vi "LoadTree2.vi"(8 "error in":errorcluster, 10 "File Path Control":path, 11 "TreeControl reference":refnum<vi>) -> (0 "error out":errorcluster)   [LabVIEW 2014]
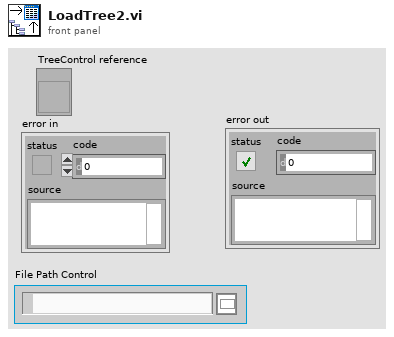
[diagram p1: front panel]
types:
  T1 = cluster{"Left Cell String":string, "Child Text":string[], "Child Tag":string, "Item Indent":i32, "Child Only?":bool, "Glyph Index":i32}[]
  T2 = cluster{"Left Cell String":string, "Child Text":string[], "Child Tag":string, "Item Indent":i32, "Child Only?":bool, "Glyph Index":i32}
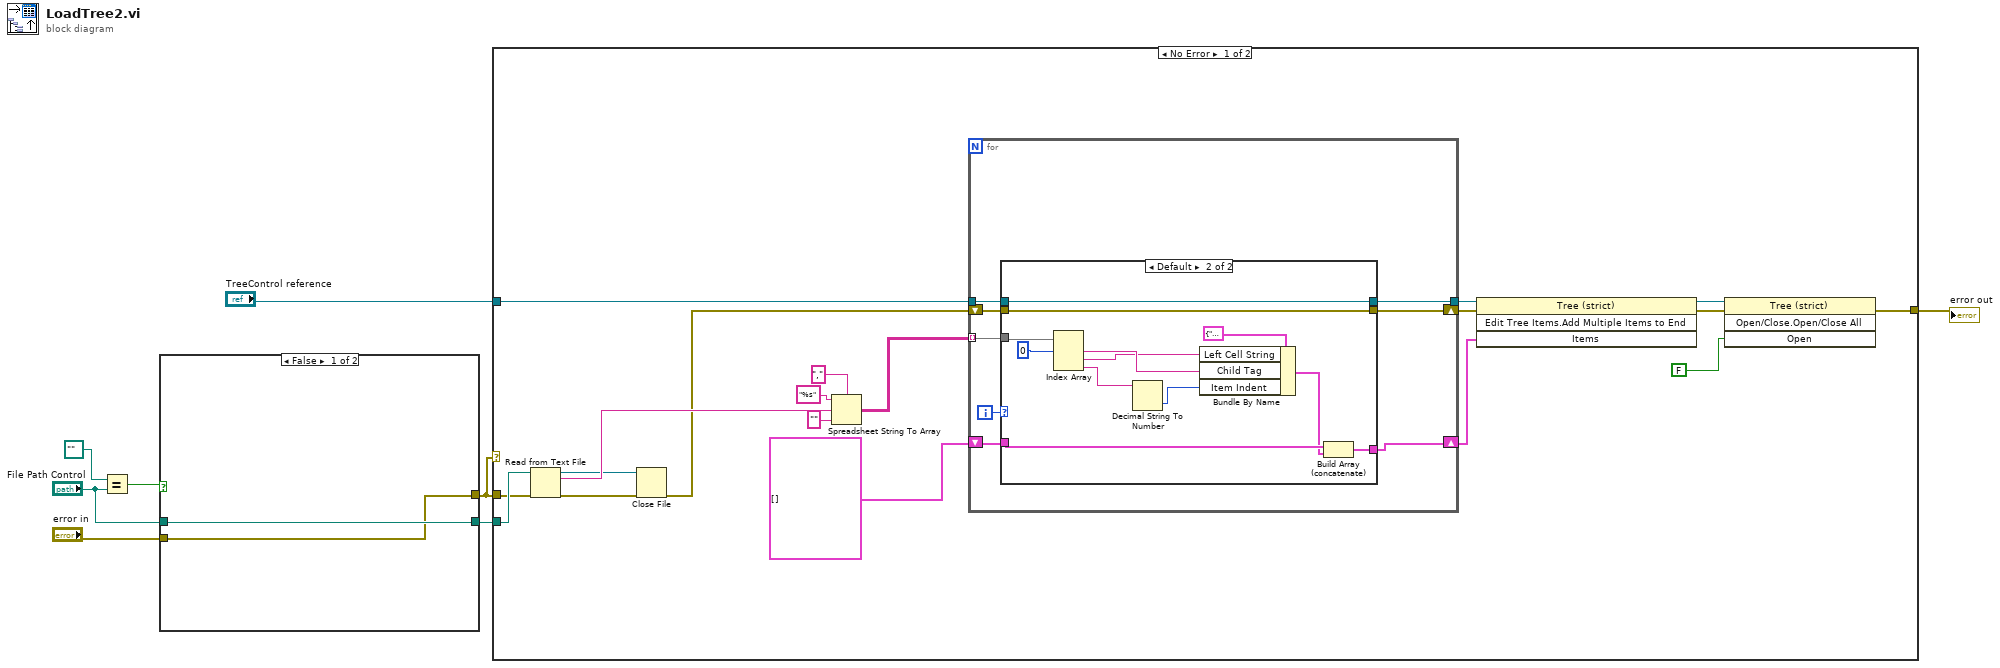
[diagram p0: block diagram]
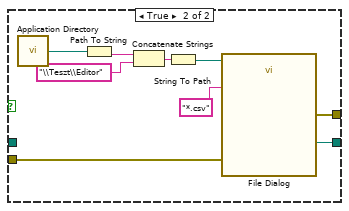
[diagram p2: hidden frame]
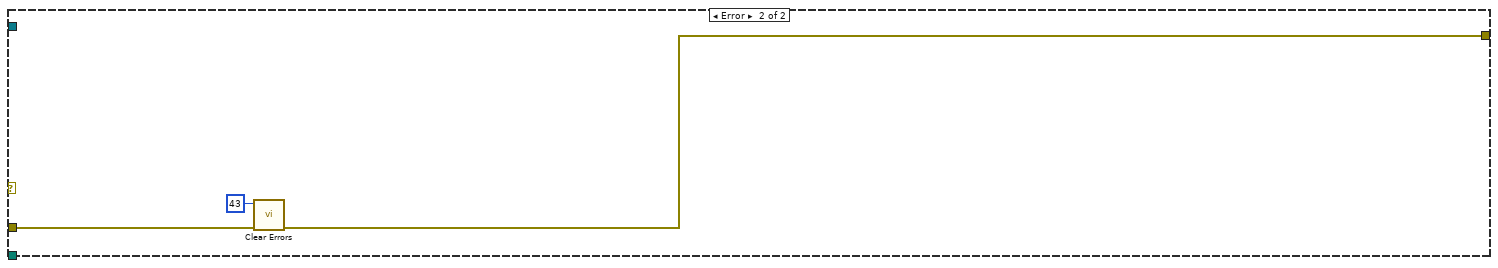
[diagram p4: hidden frame]
diagram:
  n1 = Equal?(x=path "" ("y"), y="File Path Control") -> (x = y?=w3:bool)
  n2 = case shown="False" w3 {
    tunnel: [w10 w13] -> w7
    tunnel: [w9 w12] -> w5
    tunnel: "File Path Control" -> [w10 _]
    tunnel: "error in" -> [w9 w11]
    frame False {
    }
    frame True {
      n3 = call <vilib>:"Application Directory.vi"() -> ("Application Directory"=w14:path)
      n4 = Path To String(path=w14) -> (string=w18:string)
      n5 = Concatenate Strings(w18, "\\Teszt\\Editor" ("prompt (Choose or enter file path)")) -> (w17:string)
      n6 = String To Path(string=w17) -> (path=w15:path)
      n7 = call "File Dialog"("start path"=w15, "error in"=w11, "pattern (all files)"="*.csv") -> ("selected path"=w13:path, "error out"=w12:errorcluster)  [unwired: 9 in, 2 out]
    }
  }
  n8 = case shown="No Error" w5 {
    tunnel: "TreeControl reference" -> [w24 _]
    tunnel: w7 -> [w33 _]
    tunnel: w5 -> [w32 w64]
    tunnel: [w22 w63] -> w6
    frame No Error {
      n9 = Read from Text File(file (use dialog)=w33, error in=w32) -> (refnum out=w36:refnum<file>, text=w37:string, error out=w35:errorcluster)  [unwired: 1 in, 2 out]
      n10 = Close File(refnum=w36, error in=w35) -> (error out=w25:errorcluster)  [unwired: 1 out]
      n11 = Spreadsheet String To Array(delimiter (Tab)=",", format string="%s", spreadsheet string=w37, array type (2D Dbl)="") -> (array=w31:string[][])
      n12 = for {
        tunnel: w24 -> [w46]
        tunnel: w31 -> [w44] mode=indexing
        shift-right: [w45] -> w29
        shift-left: w25 -> [w43]
        tunnel: [w42] -> w30
        shift-right: [w40] -> w27
        shift-left: T1 [] -> [w41]
        i -> [w39]
        n13 = case shown="Default" w39 {
          tunnel: w46 -> [w48 w53]
          tunnel: w43 -> [w49 w54]
          tunnel: [w49 w54] -> w45
          tunnel: w44 -> [_ w59]
          tunnel: [w48 w53] -> w42
          tunnel: w41 -> [w47 w52]
          tunnel: [w47 w50] -> w40
          frame 0 {
            # "fejlécet eldobjuk"
          }
          frame Default {
            n14 = Index Array(array=w59, index #1=0 ("index")) -> (element #1=w56:string, element #2=w55:string, element #3=w60:string)  [unwired: 2 in]
            n15 = Decimal String To Number(string=w60) -> (number=w57:i32)  [unwired: 2 in, 1 out]
            n16 = Bundle By Name(cluster=T2 {"Left Cell String"="Top Level Parent", "Child Text"=[], "Child Tag"="", "Item Indent"=0, "Child Only?"=FALSE, "Glyph Index"=0} ("Item"), "Left Cell String"=w55, "Child Tag"=w56, "Item Indent"=w57) -> (w51:T2)
            n17 = Build Array (concatenate)(w52, w51) -> (w50:T1)
          }
        }
      }
      n18 = invoke on="Invoke Node" class="Tree (strict)" method="Edit Tree Items.Add Multiple Items to End"(reference=w30, error in=w29, "Items"=w27) -> (reference out=w23:refnum<vi>, error out=w21:errorcluster)  [unwired: 1 in, 2 out]
      n19 = invoke on="Invoke Node" class="Tree (strict)" method="Open/Close.Open/Close All"(reference=w23, error in=w21, "Open"=FALSE ("Open?")) -> (error out=w22:errorcluster)  [unwired: 1 in, 3 out]
    }
    frame Error {
      n20 = call <vilib>:"Clear Errors.vi"("error in (no error)"=w64, "specific error code to clear (0: all)"=43) -> ("error out"=w63:errorcluster)  [unwired: 4 in, 1 out]
    }
  }
  "error out" <- w6
